vi "calc_mean_curve.vi"(7 "plot_properties":T1={"x_axis"={"min"=nan, "max"=nan, "label"="", "scale"=enum."Default"}, "y_axis"={"min"=nan, "max"=nan, "label"="", "scale"=enum."Default"}, "y multiplier"=0.0, "alpha"=0.0, "base_tag"="", "itens_base_name"="", "graph_title"="", "plot_names"=[], "plot_all"=FALSE}, 11 "data":T4[](array[typedef])) -> (1 "valid":bool, 2 "plots":cluster{"Ramp Pattern":dbl[], "Array":dbl[]}[](array[cluster]), 3 "mean_plot":cluster{"Ramp Pattern":dbl[], "Array":dbl[]})   [LabVIEW 2016]
uses:
  data_mean_plot.ctl
  plot_props.ctl
  axis_props.ctl
  <vilib>/Heliosphere Research LLC/Advanced Plotting Toolkit/api_core/NewPlotScales.ctl
  <vilib>/Analysis/baseanly.llb/Mean (DBL).vi
  <vilib>/Analysis/1siggen.llb/Ramp Pattern by Delta.vi
  <vilib>/Analysis/NI_AALBase.lvlib
  <vilib>/Heliosphere Research LLC/Advanced Plotting Toolkit/Advanced Plotting Toolkit.lvlib
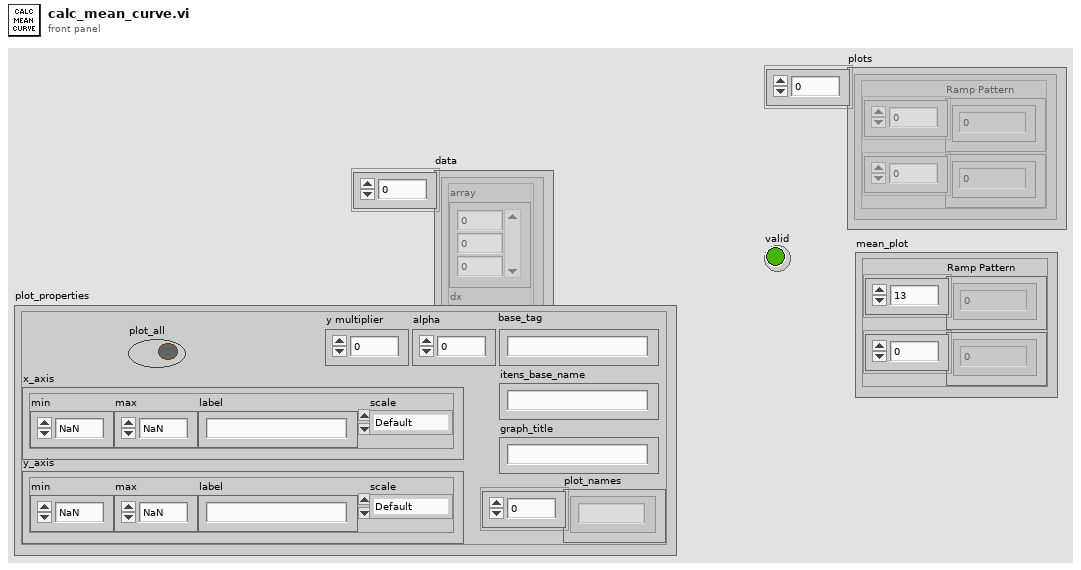
[diagram p1: front panel]
types:
  T1 = typedef "plot_props.ctl" = cluster{"x_axis":T2, "y_axis":T2, "y multiplier":dbl, "alpha":dbl, "base_tag":string, "itens_base_name":string, "graph_title":string, "plot_names":string[], "plot_all":bool}
  T2 = typedef "axis_props.ctl" = cluster{"min":dbl, "max":dbl, "label":string, "scale":T3}
  T3 = typedef "Advanced Plotting Toolkit.lvlib/NewPlotScales.ctl" = enum16{"Default", "Linear", "Log", "Symlog"}
  T4 = typedef "data_mean_plot.ctl" = cluster{"array":dbl[], "dx":dbl, "x0":dbl}
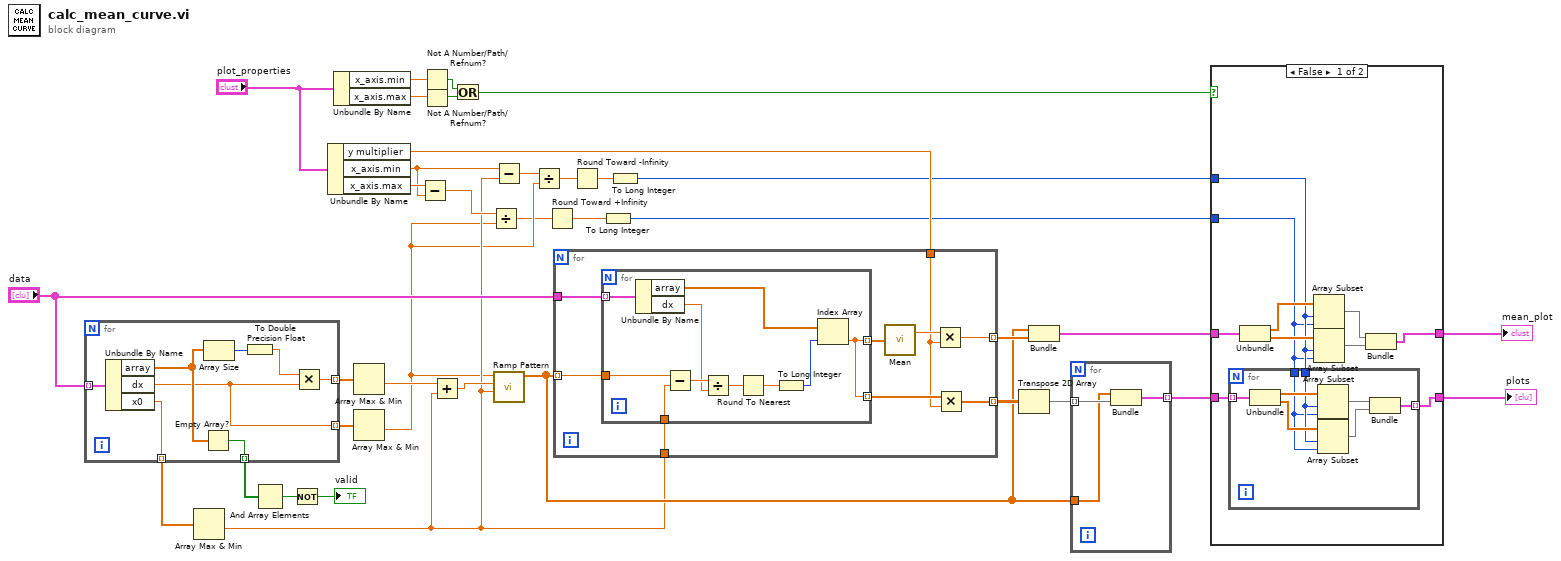
[diagram p0: block diagram]
diagram:
  n1 = for {
    tunnel: [w42] -> w36 mode=indexing
    tunnel: [w38] -> w35 mode=indexing
    tunnel: [w41] -> w28 mode=indexing
    tunnel: "data" -> [w40] mode=indexing
    tunnel: [w37] -> w24 mode=indexing
    n2 = Unbundle By Name(w40) -> ("array"=w39:dbl[], "dx"=w38:dbl, "x0"=w37:dbl)
    n3 = Empty Array?(array=w39) -> (empty?=w41:bool)
    n4 = Array Size(array=w39) -> (size(s)=w44:i32)
    n5 = To Double Precision Float(number=w44) -> (double precision float=w43:dbl)
    n6 = Multiply(x=w43, y=w38) -> (x*y=w42:dbl)
  }
  n7 = Array Max & Min(array=w24) -> (min value=w19:dbl)  [unwired: 3 out]
  n8 = And Array Elements(Boolean array=w28) -> (logical AND=w27:bool)
  n9 = Not(x=w27) -> (.not. x?=→"valid":bool)
  n10 = Unbundle By Name("plot_properties") -> ("y multiplier"=w23:dbl, "x_axis.min"=w20:dbl, "x_axis.max"=w22:dbl)
  n11 = Unbundle By Name("plot_properties") -> ("x_axis.min"=w15:dbl, "x_axis.max"=w14:dbl)
  n12 = Array Max & Min(array=w36) -> (min value=w34:dbl)  [unwired: 3 out]
  n13 = Array Max & Min(array=w35) -> (min value=w17:dbl)  [unwired: 3 out]
  n14 = Subtract(x=w22, y=w20) -> (x-y=w21:dbl)
  n15 = Not A Number/Path/Refnum?(number/path/refnum=w15) -> (NaN/Path/Refnum?=w12:bool)
  n16 = Not A Number/Path/Refnum?(number/path/refnum=w14) -> (NaN/Path/Refnum?=w13:bool)
  n17 = Add(x=w34, y=w19) -> (x+y=w29:dbl)
  n18 = Or(x=w12, y=w13) -> (x .or. y?=w6:bool)
  n19 = Divide(x=w21, y=w17) -> (x/y=w10:dbl)
  n20 = Subtract(x=w20, y=w19) -> (x-y=w18:dbl)
  n21 = call-poly <vilib>:"Ramp Pattern.vi"("start"=w19, "end"=w29, "delta"=w17) -> ("Ramp Pattern"=w30:dbl[])  [unwired: 6 in, 2 out]
  n22 = Divide(x=w18, y=w17) -> (x/y=w11:dbl)
  n23 = Round Toward +Infinity(x=w10) -> (ceil(x): smallest int >= x=w8:dbl)
  n24 = for {
    tunnel: w30 -> [w52] mode=indexing
    tunnel: "data" -> [w53]
    tunnel: [w47] -> w33 mode=indexing
    tunnel: [w49] -> w31 mode=indexing
    tunnel: w23 -> [w46]
    tunnel: w19 -> [w45]
    n25 = for {
      tunnel: w53 -> [w56] mode=indexing
      tunnel: w52 -> [w59]
      tunnel: [w60] -> w51 mode=indexing
      tunnel: [w60] -> w48 mode=indexing
      tunnel: w45 -> [w58]
      n26 = Unbundle By Name(w56) -> ("array"=w55:dbl[], "dx"=w54:dbl)
      n27 = Subtract(x=w59, y=w58) -> (x-y=w57:dbl)
      n28 = Divide(x=w57, y=w54) -> (x/y=w63:dbl)
      n29 = Round To Nearest(number=w63) -> (nearest integer value=w62:dbl)
      n30 = To Long Integer(number=w62) -> (32bit integer=w61:i32)
      n31 = Index Array(array=w55, index=w61) -> (element=w60:dbl)
    }
    n32 = call-poly <vilib>:"Mean.vi"("X"=w51) -> ("mean"=w50:dbl)  [unwired: 1 out]
    n33 = Multiply(x=w50, y=w46) -> (x*y=w49:dbl)
    n34 = Multiply(x=w48, y=w46) -> (x*y=w47:dbl[])
  }
  n35 = Round Toward -Infinity(1:w11) -> (0:w9:dbl)
  n36 = To Long Integer(number=w8) -> (32bit integer=w1:i32)
  n37 = To Long Integer(number=w9) -> (32bit integer=w2:i32)
  n38 = Transpose 2D Array(2D array=w33) -> (transposed array=w32:dbl[][])
  n39 = Bundle("Ramp Pattern"=w30, w31) -> (w3:cluster{"Ramp Pattern":dbl[], dbl[]})  [unwired: 1 in]
  n40 = for {
    tunnel: w32 -> [w66] mode=indexing
    tunnel: w30 -> [w65]
    tunnel: [w64] -> w7 mode=indexing
    n41 = Bundle("Ramp Pattern"=w65, w66) -> (w64:cluster{"Ramp Pattern":dbl[], dbl[]})  [unwired: 1 in]
  }
  n42 = case shown="False" w6 {
    tunnel: w7 -> [w73 w86]
    tunnel: [w67 w86] -> w5
    tunnel: [w68 w85] -> w4
    tunnel: w3 -> [w76 w85]
    tunnel: w2 -> [w72 _]
    tunnel: w1 -> [w71 _]
    frame False {
      n43 = for {
        tunnel: w73 -> [w84] mode=indexing
        tunnel: w72 -> [w81]
        tunnel: w71 -> [w80]
        tunnel: [w77] -> w67 mode=indexing
        n44 = Unbundle(w84) -> ("Ramp Pattern"=w83:dbl[], w82:dbl[])
        n45 = Array Subset(array=w83, index=w81, length=w80) -> (w79:dbl[])
        n46 = Array Subset(array=w82, index=w81, length=w80) -> (w78:dbl[])
        n47 = Bundle(w79, w78) -> (w77:cluster{dbl[], dbl[]})  [unwired: 1 in]
      }
      n48 = Unbundle(w76) -> ("Ramp Pattern"=w75:dbl[], w74:dbl[])
      n49 = Array Subset(array=w75, index=w72, length=w71) -> (w69:dbl[])
      n50 = Array Subset(array=w74, index=w72, length=w71) -> (w70:dbl[])
      n51 = Bundle(w69, w70) -> (w68:cluster{dbl[], dbl[]})  [unwired: 1 in]
    }
    frame True {
    }
  }
  "plots" <- w5
  "mean_plot" <- w4
